vi "Query Slits.vi"(8 "error in (no error)":errorcluster, 11 "VISA resource name":refnum<visa-resource-name>) -> (0 "error out":errorcluster, 1 "CURRENT S2 WIDTH":dbl[unit] min=0.0 max=0.005000000000000002 step=1.0000000000000004e-06, 2 "CURRENT S1 WIDTH":dbl[unit] min=0.0 max=0.005000000000000002 step=1.0000000000000004e-06, 3 "VISA resource name out":refnum<visa-resource-name>, 4 "CURRENT S3 WIDTH":dbl[unit] min=0.0 max=0.005000000000000002 step=1.0000000000000004e-06)   [LabVIEW 2023, in "Digikrom DK24x.lvlib"]
doc: "Returns the current entrance, exit (and for DK242) middle slit width in microns."
uses:
  Digikrom DK24x.lvlib
  Private/Command.ctl
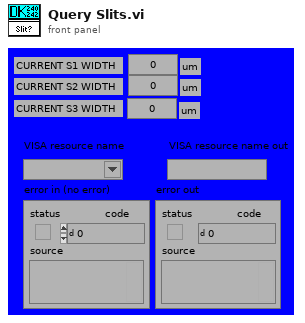
[diagram p1: front panel]
types:
  T1 = typedef "Digikrom DK24x.lvlib/Command.ctl" = u8
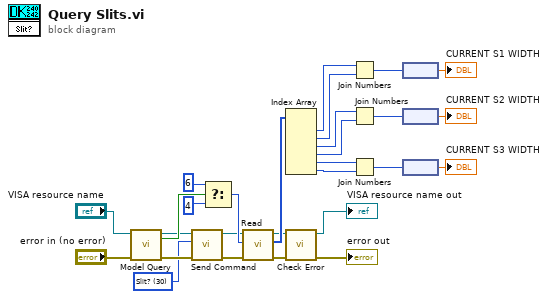
[diagram p0: block diagram]
diagram:
  w1 = T1 30 items=["Cancel"=24, "Clear"=25, "CSR"=28, "Echo"=27, "Filter"=15, "Gcal"=18, "Goto"=16, "Grtid?"=19, "Grtsel"=26, "NOVRAM Read"=56, "NOVRAM Write"=59, "Reset"=255, "Scan"=12, "Scan Up"=9, "Scan Down"=3, "Serial?"=33, "Slew Up"=8, "Slew Down"=2, "Slit Reset"=43, "Slit?"=30, "Sltadj"=14, "Speed"=13, "Sspeed?"=21, "Step Down"=1, "Step Up"=7, "S1adj"=31, "S2adj"=32, "S3adj"=34, "S1cal"=22, "S2cal"=23, "S3cal"=35, "Test"=17, "Type"=57, "Wave?"=29, "Zero"=52] ("Command")
  n1 = call "Model Query.vi"("error in (no error)"="error in (no error)", "VISA resource name"="VISA resource name") -> ("error out"=w4:errorcluster, "Is DK242?"=w8:bool, "VISA resource name out"=w5:refnum<visa-resource-name>)  [unwired: 3 in, 4 out]
  n2 = call "Send Command.vi"("error in (no error)"=w4, "Command"=w1, "VISA resource name"=w5) -> ("error out"=w3:errorcluster, "VISA resource name out"=w2:refnum<visa-resource-name>)  [unwired: 7 out]
  n3 = Select(t=u8 6, s=w8, f=u8 4) -> (s? t:f=w10:u8)
  n4 = call "Read.vi"("error in (no error)"=w3, "response size"=w10, "VISA resource name"=w2) -> ("error out"=w18:errorcluster, "response array"=w24:u8[], "VISA resource name out"=w19:refnum<visa-resource-name>)  [unwired: 6 out]
  n5 = Index Array(array=w24) -> (element #1=w22:u8, element #2=w23:u8, element #3=w25:u8, element #4=w26:u8, element #5=w13:u8, element #6=w12:u8)  [unwired: 6 in]
  n6 = call "Check Error.vi"("error in"=w18, "VISA resource name in"=w19) -> ("error out"=→"error out":errorcluster, "VISA resource name out"=→"VISA resource name out":refnum<visa-resource-name>)  [unwired: 1 in, 7 out]
  n7 = Join Numbers(hi=w22, lo=w23) -> ((hi.lo)=w14:u16)
  n8 = Join Numbers(hi=w25, lo=w26) -> ((hi.lo)=w16:u16)
  n9 = Join Numbers(hi=w13, lo=w12) -> ((hi.lo)=w28:u16)
  n10 = node(w14) -> (→"CURRENT S1 WIDTH":dbl[unit])
  n11 = node(w16) -> (→"CURRENT S2 WIDTH":dbl[unit])
  n12 = node(w28) -> (→"CURRENT S3 WIDTH":dbl[unit])
